vi "KINECTAverage.vi"(10 "Min":dbl, 11 "Max":dbl) -> (2 "Range/2":dbl, 3 "Average":dbl)   [LabVIEW 2011]
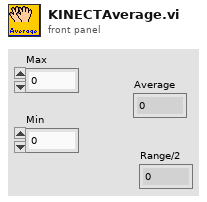
[diagram p1: front panel]
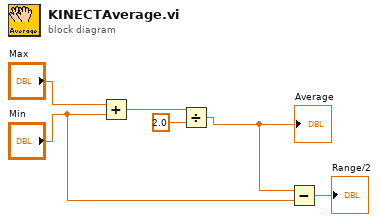
[diagram p0: block diagram]
diagram:
  n1 = Add(x="Max", y="Min") -> (x+y=w5:dbl)
  n2 = Divide(x=w5, y=2.0) -> (x/y=w3:dbl)
  "Average" <- w3
  n3 = Subtract(x=w3, y="Min") -> (x-y=→"Range/2":dbl)
